vi "Error_AddAdditionalInformation.vi"(6 "Additional Info":string, 8 "Error In":errorcluster) -> (0 "Error Out":errorcluster)   [LabVIEW 2020, in "hse-misc.lvlib"]
doc: "Adds <b>Additional Info</b> to the source of <b>Error In</b>\n\n\n\n____\nHAMPEL SOFTWARE ENGINEERING v3.8.0 (2023-12-18 14:41)"
uses:
  hse-misc.lvlib
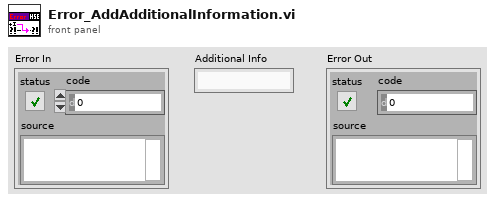
[diagram p1: front panel]
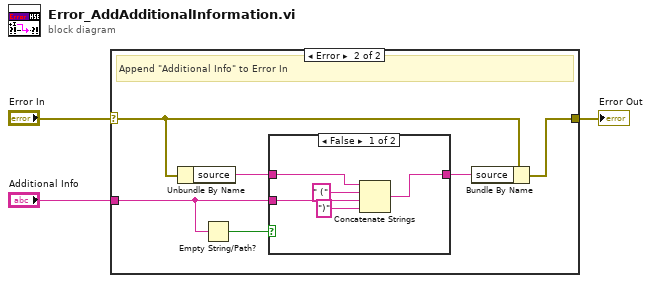
[diagram p0: block diagram]
diagram:
  n1 = case shown="Error" "Error In" {
    selector: "Error In" -> [w4 w6]
    tunnel: [w4 w5] -> w3
    tunnel: "Additional Info" -> [_ w9]
    frame No Error {
      # "Do nothing"
    }
    frame Error {
      # "Append \"Additional Info\" to Error In"
      n2 = Unbundle By Name(w6) -> ("source"=w7:string)
      n3 = Empty String/Path?(string/path=w9) -> (empty?=w10:bool)
      n4 = case shown="False" w10 {
        tunnel: w9 -> [w15 _]
        tunnel: [w11 w16] -> w8
        tunnel: w7 -> [w12 w16]
        frame False {
          n5 = Concatenate Strings(w12, " (" ("string"), w15, ")" ("string")) -> (w11:string)
        }
        frame True {
        }
      }
      n6 = Bundle By Name(cluster=w6, "source"=w8) -> (w5:errorcluster)
    }
  }
  "Error Out" <- w3
